vi "例4-33.vi"() -> ()   [LabVIEW 2019]
uses:
  <vilib>/Waveform/DWDTOps.llb/DWDT Analog to Digital.vi
panel:
  out "二进制表示法":digitaldata
  in  "数字":dbl[](array[numeric])
  out "数字波形图":digitalwaveform(graph)
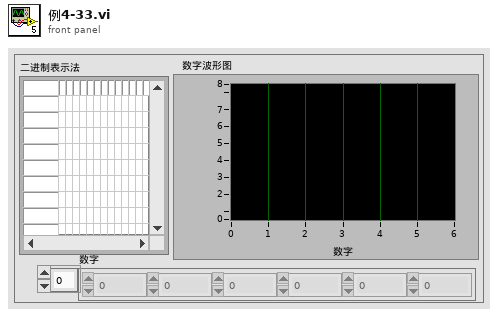
[diagram p1: front panel]
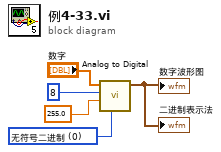
[diagram p0: block diagram]
diagram:
  w2 = u16 0 items=["无符号二进制", "二进制偏移量", "二进制补码"] ("data format (offset binary)")
  n1 = call-poly <vilib>:"Analog to Digital.vi"("data format (offset binary)"=w2, "full-scale range (pk-pk)"=255.0, "resolution (16 bit)"=8, "analog waveform"="数字") -> ("digital waveform"=→"数字波形图" →"二进制表示法":digitalwaveform)  [unwired: 4 in, 3 out]
